vi "getOrAlloc.vi"(8 "error in (no error)":errorcluster, 9 "requested size":u64, 10 "current buffer":T1) -> (0 "error out":errorcluster, 1 "is locked":bool, 2 "output buffer":T1)   [LabVIEW 2016]
uses:
  private/vis/BufferStruct.ctl
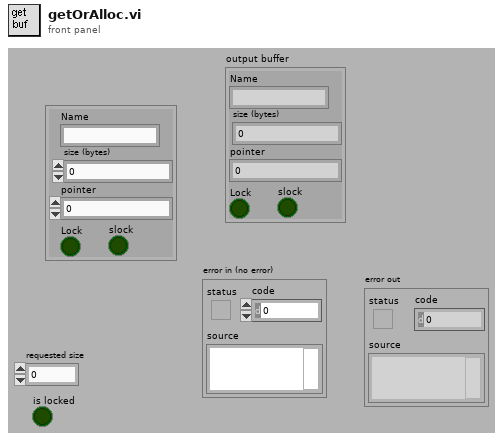
[diagram p1: front panel]
types:
  T1 = typedef "BufferStruct.ctl" = cluster{"Name":string, "size (bytes)":u64, "pointer":u64, "Lock":bool, "slock":bool}
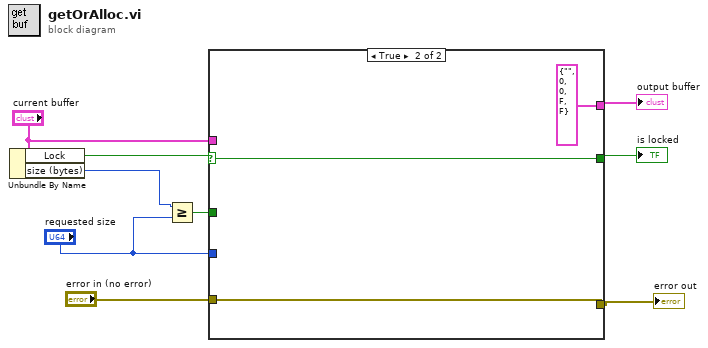
[diagram p0: block diagram]
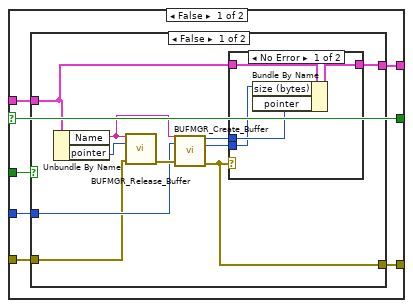
[diagram p2: hidden frame]
diagram:
  n1 = Unbundle By Name("current buffer") -> ("Lock"=w6:bool, "size (bytes)"=w9:u64)
  n2 = Greater Or Equal?(x=w9, y="requested size") -> (x >= y?=w8:bool)
  n3 = case shown="True" w6 {
    selector: w6 -> [w14 w36]
    tunnel: w8 -> [w16 _]
    tunnel: "current buffer" -> [w15 _]
    tunnel: [w14 w36] -> w5
    tunnel: [w12 T1 {"Name"="", "size (bytes)"=0, "pointer"=0, "Lock"=FALSE, "slock"=FALSE} ("current buffer")] -> w4
    tunnel: "requested size" -> [w13 _]
    tunnel: "error in (no error)" -> [w11 w35]
    tunnel: [w10 w35] -> w1
    frame False {
      n4 = case shown="False" w16 {
        tunnel: w15 -> [w18 w33]
        tunnel: w13 -> [w23 _]
        tunnel: [w17 w33] -> w12
        tunnel: w11 -> [w20 w32]
        tunnel: [w19 w32] -> w10
        frame False {
          n5 = Unbundle By Name(w18) -> ("Name"=w24:string, "pointer"=w25:u64)
          n6 = call "BUFMGR_Release_Buffer.vi"("Buffer Name"=w24, "buffer in"=w25, "error in (no error)"=w20) -> ("error out"=w26:errorcluster)  [unwired: 12 out]
          n7 = call "BUFMGR_Create_Buffer.vi"("Buffer Name"=w24, "Size in Bytes"=w23, "error in (no error)"=w26) -> ("pointer to buff"=w22:u64, "Size in Bytes out"=w21:u64, "error out"=w19:errorcluster)  [unwired: 10 out]
          n8 = case shown="No Error" w19 {
            tunnel: w18 -> [w30 w31]
            tunnel: w22 -> [w29 _]
            tunnel: w21 -> [w28 _]
            tunnel: [w27 w31] -> w17
            frame No Error {
              n9 = Bundle By Name(cluster=w30, "size (bytes)"=w28, "pointer"=w29) -> (w27:T1)
            }
            frame Error {
            }
          }
        }
        frame True {
        }
      }
    }
    frame True {
    }
  }
  "is locked" <- w5
  "output buffer" <- w4
  "error out" <- w1
